vi "moje2.vi"() -> ()   [LabVIEW 2015]
uses:
  <vilib>/DAQmx/read.llb/DAQmx Read (Analog DBL 1Chan 1Samp).vi
  <vilib>/DAQmx/create/channels.llb/DAQmx Create Channel (AI-Voltage-Basic).vi
  <vilib>/DAQmx/configure/timing.llb/DAQmx Timing (Sample Clock).vi
  <vilib>/DAQmx/miscellaneous.llb/DAQmx Fill In Error Info.vi
panel:
  out "data":dbl format="%0.2f"
  in  "Czestotliwosc":dbl=1000.0 format="%0.2f"
  in  "physical channels":tag
  in  "error in":errorcluster
  in  "stop":bool
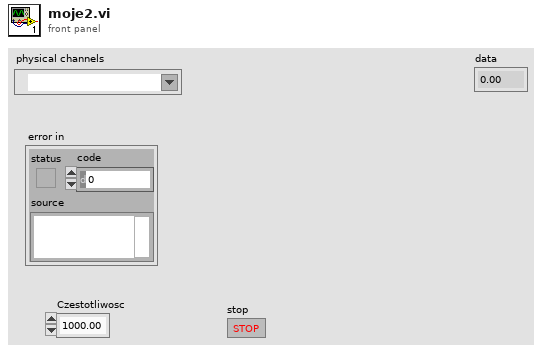
[diagram p1: front panel]
types:
  T1 = enum16{"open", "replace", "create", "open or create", "replace or create", "replace or create with confirmation"}
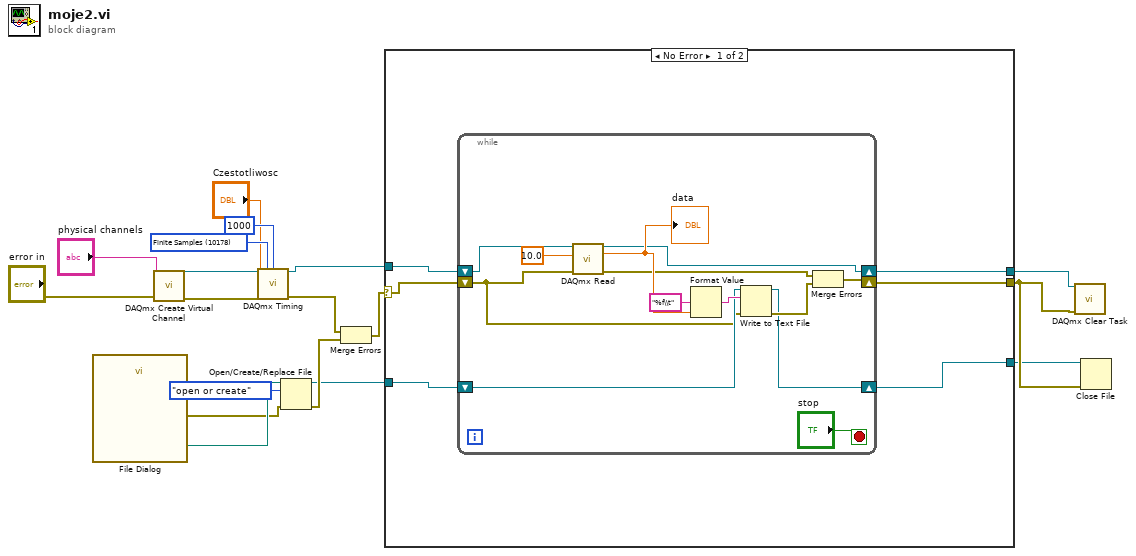
[diagram p0: block diagram]
diagram:
  w14 = 10178 items=["Finite Samples"=10178, "Continuous Samples"=10123, "Hardware Timed Single Point"=12522] ("sample mode")
  n1 = call "File Dialog"() -> ("selected path"=w11:path, "error out"=w10:errorcluster)  [unwired: 12 in, 2 out]
  n2 = call-poly <vilib>:"DAQmx Create Virtual Channel.vi"("physical channels"="physical channels", "error in"="error in") -> ("task out"=w15:refnum<k21>, "error out"=w16:errorcluster)  [unwired: 12 in]
  n3 = call-poly <vilib>:"DAQmx Timing.vi"("task/channels in"=w15, "sample mode"=w14, "samples per channel"=1000, "rate"="Czestotliwosc", "error in"=w16) -> ("task out"=w5:refnum<k21>, "error out"=w8:errorcluster)  [unwired: 9 in]
  n4 = Open/Create/Replace File(file path (use dialog)=w11, error in=w10, operation (0:open)=T1."open or create") -> (refnum out=w6:refnum<file>, error out=w9:errorcluster)  [unwired: 3 in, 1 out]
  n5 = Merge Errors(w8, w9) -> (w7:errorcluster)
  n6 = case shown="No Error" w7 {
    selector: w7 -> [w22 w39]
    tunnel: w6 -> [w24 w38]
    tunnel: w5 -> [w23 w40]
    tunnel: [w21 w39] -> w3
    tunnel: [w20 w40] -> w4
    tunnel: [w19 w38] -> w2
    frame No Error {
      n7 = while {
        shift-right: [w25] -> w20
        shift-left: w23 -> [w36]
        shift-right: [w26] -> w19
        shift-left: w24 -> [w31]
        shift-right: [w29] -> w21
        shift-left: w22 -> [w30]
        stop <- "stop" stop-if-true
        n8 = call-poly <vilib>:"DAQmx Read.vi"("task/channels in"=w36, "timeout"=10.0, "error in"=w30) -> ("task out"=w25:refnum<k21>, "data"=w33:dbl, "error out"=w27:errorcluster)  [unwired: 10 in]
        "data" <- w33
        n9 = Format Value(format string="%f\\t", value (0)=w33) -> (output string=w34:string)  [unwired: 1 in]
        n10 = Write to Text File(file (use dialog)=w31, text=w34, error in=w30) -> (refnum out=w26:refnum<file>, error out=w28:errorcluster)  [unwired: 1 in, 1 out]
        n11 = Merge Errors(w27, w28) -> (w29:errorcluster)
      }
    }
    frame Error {
    }
  }
  n12 = call <vilib>:"DAQmx Clear Task.vi"("task in"=w4, "error in"=w3) -> ()  [unwired: 13 in, 1 out]
  n13 = Close File(refnum=w2, error in=w3) -> ()  [unwired: 2 out]
